vi "NI6071E.SaveDAQData.vi"(0 "i ref in":refnum<vi>, 4 "timeout ms (60000)":i32=60000, 5 "error in (no error)":errorcluster) -> (14 "i ref out":refnum<vi>, 19 "error out":errorcluster)   [LabVIEW 2014, in "NI6071E.lvlib"]
uses:
  NI6071E.lvlib
  NI6071ECommandCluster.ctl
  NI6071ECommand.ctl
panel:
  in  "PPMA Command":T1=enum."ConfigureDAQ"
  in  "PPMA Command Cluster":T2
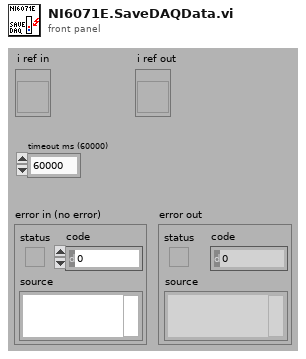
[diagram p1: front panel]
types:
  T1 = typedef "NI6071E.lvlib/NI6071ECommand.ctl" = enum16{"Ping", "Reset", "ConfigureDAQ", "StartDAQ", "StopDAQ", "GetDAQStatus", "ReadData", "SaveData", "CloseConnection"}
  T2 = typedef "NI6071E.lvlib/NI6071ECommandCluster.ctl" = cluster{"Command":string, "Data":string, "error out":errorcluster}
  T3 = typedef "NI6071E.lvlib/NI6071E.i attribute.ctl" = cluster{"NI6071E Server":string, "Port":u16, "NI6071E Config":T4, "NI6071E Start":T5, "Waveforms":waveform(dbl)[], "RT Error":errorcluster, "NI6071E Read":T6, "connection ID":refnum<k5>, "DAQ Status":string, "device (1)":i16, "DAQ Status Service ID":i32}
  T4 = typedef "NI6071E.lvlib/NI6071EConfig.ctl" = cluster{"device (1)":i16, "channels (0)":tag[], "buffer size (1000 scans)":i32, "[number of buffers] (1)":i32, "measurement mode structure":cluster{"measurement mode":u16, "reserved":u32}, "input limits (no change)":cluster{"high limit (0.0)":sgl, "low limit (0.0)":sgl}[], "coupling & input config (no change:0)":cluster{"coupling (no change:0)":enum16{"no change", "DC", "AC", "GND", "internal ref."}, "input config (no change:0)":u16}[]}
  T5 = typedef "NI6071E.lvlib/NI6071EStart.ctl" = cluster{"scan rate (40000 scans/sec)":sgl, "trigger type (analog)":enum16{"no trigger", "analog", "digital A", "digital A & B", "scan clock gate"}, "edge or slope \n(rising)":enum16{"no change", "rising", "falling"}, "number of buffers to acquire (1)":i32, "analog chan (PFI0) & level (2.00)":cluster{"trigger channel (empty)":string, "level (0.0)":sgl}, "[additional trig params]":cluster{"hysteresis (0.0)":sgl, "coupling (no change:0)":enum16{"no change", "DC", "AC"}, "delay (0 sec)":sgl, "skip count (0)":i32, "time limit (0 sec)":sgl}}
  T6 = typedef "NI6071E.lvlib/NI6071ERead.ctl" = cluster{"time limit in sec (-1:auto calculate)":sgl, "number of scans to read (-1:all)":i32}
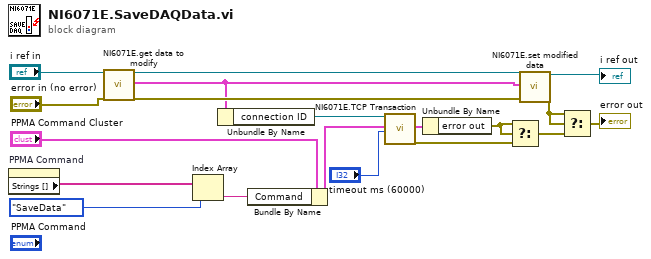
[diagram p0: block diagram]
diagram:
  n1 = property on="PPMA Command" class="Enum (strict)"() -> ("Strings []"=w9:string[])  [unwired: 2 in, 2 out]
  n2 = call "NI6071E.get data to modify.vi"("i ref in"="i ref in", "error in (no error)"="error in (no error)") -> ("i ref out"=w16:refnum<vi>, "i attribute"=w1:T3, "error out"=w17:errorcluster)  [unwired: 14 in, 1 out]
  n3 = Index Array(array=w9, index=NI6071ECommand."SaveData" ("PPMA Command")) -> (element=w7:string)
  n4 = Unbundle By Name(w1) -> ("connection ID"=w12:refnum<k5>)
  n5 = Bundle By Name(cluster="PPMA Command Cluster", "Command"=w7) -> (w10:T2)
  n6 = call "NI6071E.TCP Transaction.vi"("connection ID in"=w12, "NI6071E Command Cluster"=w10, "timeout ms (25000)"="timeout ms (60000)") -> ("NI6071E Response"=w5:T2, "error out"=w3:errorcluster)  [unwired: 14 in, 1 out]
  n7 = Unbundle By Name(w5) -> ("error out"=w4:errorcluster)
  n8 = Select(t=w4, s=w4, f=w3) -> (s? t:f=w2:errorcluster)
  n9 = call "NI6071E.set modified data.vi"("i ref in"=w16, "i attribute"=w1, "error in (no error)"=w17) -> ("i ref out"=→"i ref out":refnum<vi>, "error out"=w14:errorcluster)  [unwired: 15 in]
  n10 = Select(t=w14, s=w14, f=w2) -> (s? t:f=→"error out":errorcluster)
